vi "Set Attribute.vi"(8 "error in (no error)":errorcluster, 9 "Data to set":refnum<class "Data.lvclass">, 10 "Name":string, 11 "Variant in":refnum<class "Variant.lvclass">) -> (0 "error out":errorcluster, 2 "Replaced?":bool, 3 "Variant out":refnum<class "Variant.lvclass">)   [LabVIEW 2020, in "Data.lvlib" / "Variant.lvclass"]
doc: "Set an attribute on the variant."
uses:
  Variant.lvclass
  Data.lvclass
  Variant.lvclass/Variant.ctl
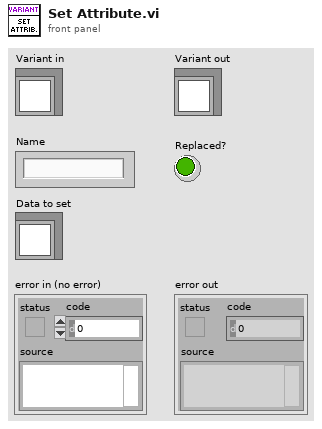
[diagram p1: front panel]
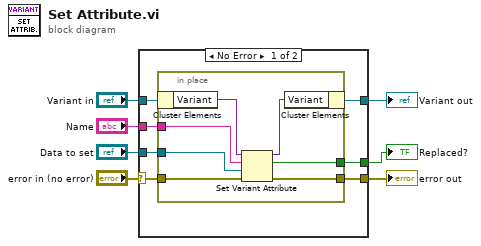
[diagram p0: block diagram]
diagram:
  n1 = case shown="No Error" "error in (no error)" {
    selector: "error in (no error)" -> [w12 w23]
    tunnel: [w11 w23] -> w6
    tunnel: [w13 w22] -> w4
    tunnel: "Variant in" -> [w14 w22]
    tunnel: "Data to set" -> [w10 _]
    tunnel: "Name" -> [w9 _]
    tunnel: [w8 _] -> w1
    frame No Error {
      n2 = in-place {
        in-place-border: w12 -> [w19]
        in-place-border: [w18] -> w11
        in-place-border: w10 -> [w17]
        in-place-border: w9 -> [w16]
        in-place-border: [w15] -> w8
        n3 = in-place-cluster #1(w14) -> ("Variant"=w21:variant)
        n4 = Set Variant Attribute(Variant=w21, name=w16, value=w17, error in=w19) -> (Variant out=w20:variant, replaced=w15:bool, error out=w18:errorcluster)
        n5 = in-place-cluster #1("Variant"=w20) -> (w13:refnum<class "Variant.lvclass">)
      }
    }
    frame Error {
    }
  }
  "error out" <- w6
  "Variant out" <- w4
  "Replaced?" <- w1
